vi "Parent Main Operation.vi"(8 "error in (no error)":errorcluster, 11 "Node Actor in":refnum<class "Node Actor.lvclass">) -> (0 "error out":errorcluster, 3 "Node Actor out":refnum<class "Node Actor.lvclass">)   [LabVIEW 2024, in "Node Actor.lvclass"]
uses:
  Node Actor.lvclass
  Message/Message.lvclass/Message.ctl
  Message/Public Data/Read CMD Type.vi
  Message/Message.lvclass
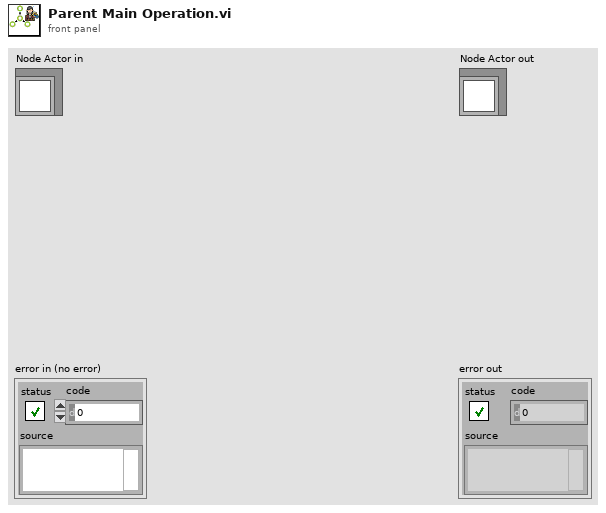
[diagram p1: front panel]
types:
  T1 = typedef "CMD Type.ctl" = enum16{"None", "General CMD", "1st CMD", "2nd CMD", "3rd CMD", "4th CMD", "5th CMD", "6th CMD", "7th CMD"}
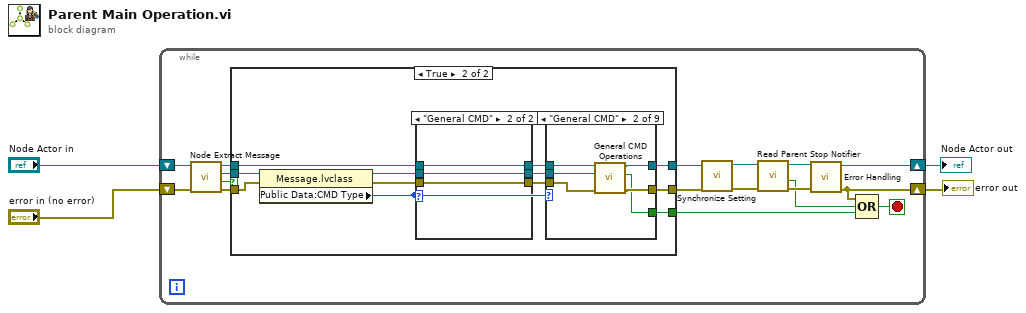
[diagram p0: block diagram]
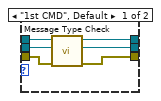
[diagram p3: hidden frame]
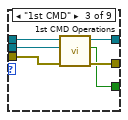
[diagram p5: hidden frame]
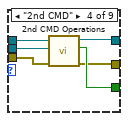
[diagram p6: hidden frame]
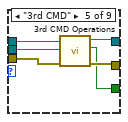
[diagram p7: hidden frame]
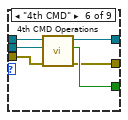
[diagram p8: hidden frame]
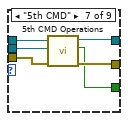
[diagram p9: hidden frame]
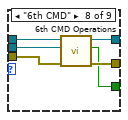
[diagram p10: hidden frame]
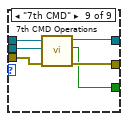
[diagram p11: hidden frame]
diagram:
  n1 = while {
    shift-right: [w13] -> w2
    shift-left: "Node Actor in" -> [w20]
    shift-right: [w6] -> w1
    shift-left: "error in (no error)" -> [w19]
    stop <- w21 stop-if-true
    n2 = call-dynamic "Node Extract Message.vi"("error in (no error)"=w19, "Node Actor in"=w20) -> ("error out"=w16:errorcluster, "Valid"=w14:bool, "Message Out"=w17:refnum<class "Message.lvclass">, "Node Actor out"=w18:refnum<class "Node Actor.lvclass">)  [unwired: 6 in]
    n3 = case shown="True" w14 {
      tunnel: [w22 w35] -> w11
      tunnel: w18 -> [w23 w27]
      tunnel: w17 -> [_ w32]
      tunnel: w16 -> [w22 w31]
      tunnel: [w23 w34] -> w12
      tunnel: [_ w33] -> w15
      frame False {
      }
      frame True {
        n4 = property class="Message.lvclass"(reference=w32, error in=w31) -> (reference out=w29:refnum<class "Message.lvclass">, error out=w28:errorcluster, "Public Data:CMD Type"=w30:T1)
        n5 = case shown="\"General CMD\"" w30 {
          tunnel: w29 -> [w40 w43]
          tunnel: w28 -> [w39 w42]
          tunnel: w27 -> [w41 w44]
          tunnel: [w36 w44] -> w26
          tunnel: [w37 w43] -> w25
          tunnel: [w38 w42] -> w24
          frame "1st CMD", Default {
            n6 = call-dynamic "Message Type Check.vi"("error in (no error)"=w39, "Message In"=w40, "System Actor in"=w41) -> ("error out"=w38:errorcluster, "Message Out"=w37:refnum<class "Message.lvclass">, "System Actor out"=w36:refnum<class "Node Actor.lvclass">)  [unwired: 6 in]
          }
          frame "General CMD" {
          }
        }
        n7 = case shown="\"General CMD\"" w30 {
          tunnel: w25 -> [_ w51 w57 w60 w69 w75 w81 w87 w93]
          tunnel: w26 -> [w46 w52 w58 w64 w70 w76 w82 w88 w94]
          tunnel: [w46 w48 w54 w63 w66 w73 w78 w85 w90] -> w34
          tunnel: w24 -> [w45 w50 w56 w59 w68 w74 w80 w86 w92]
          tunnel: [w45 w49 w55 w61 w67 w71 w79 w84 w91] -> w35
          tunnel: [_ w47 w53 w62 w65 w72 w77 w83 w89] -> w33
          frame "None", Default {
          }
          frame "General CMD" {
            n8 = call-dynamic "General CMD Operations.vi"("error in (no error)"=w50, "Message In"=w51, "System Actor in"=w52) -> ("error out"=w49:errorcluster, "Stop"=w47:bool, "System Actor out"=w48:refnum<class "Node Actor.lvclass">)  [unwired: 6 in]
          }
          frame "1st CMD" {
            n9 = call-dynamic "1st CMD Operations.vi"("error in (no error)"=w56, "Message In"=w57, "Node Actor in"=w58) -> ("error out"=w55:errorcluster, "Stop"=w53:bool, "Node Actor out"=w54:refnum<class "Node Actor.lvclass">)  [unwired: 6 in]
          }
          frame "2nd CMD" {
            n10 = call-dynamic "2nd CMD Operations.vi"("error in (no error)"=w59, "Message In"=w60, "System Actor in"=w64) -> ("error out"=w61:errorcluster, "Stop"=w62:bool, "System Actor out"=w63:refnum<class "Node Actor.lvclass">)  [unwired: 6 in]
          }
          frame "3rd CMD" {
            n11 = call-dynamic "3rd CMD Operations .vi"("error in (no error)"=w68, "Message In"=w69, "System Actor in"=w70) -> ("error out"=w67:errorcluster, "Stop"=w65:bool, "System Actor out"=w66:refnum<class "Node Actor.lvclass">)  [unwired: 6 in]
          }
          frame "4th CMD" {
            n12 = call-dynamic "4th CMD Operations.vi"("error in (no error)"=w74, "Message In"=w75, "System Actor in"=w76) -> ("error out"=w71:errorcluster, "Stop"=w72:bool, "System Actor out"=w73:refnum<class "Node Actor.lvclass">)  [unwired: 6 in]
          }
          frame "5th CMD" {
            n13 = call-dynamic "5th CMD Operations.vi"("error in (no error)"=w80, "Message In"=w81, "System Actor in"=w82) -> ("error out"=w79:errorcluster, "Stop"=w77:bool, "System Actor out"=w78:refnum<class "Node Actor.lvclass">)  [unwired: 6 in]
          }
          frame "6th CMD" {
            n14 = call-dynamic "6th CMD Operations .vi"("error in (no error)"=w86, "Message In"=w87, "System Actor in"=w88) -> ("error out"=w84:errorcluster, "Stop"=w83:bool, "System Actor out"=w85:refnum<class "Node Actor.lvclass">)  [unwired: 6 in]
          }
          frame "7th CMD" {
            n15 = call-dynamic "7th CMD Operations.vi"("error in (no error)"=w92, "Message In"=w93, "System Actor in"=w94) -> ("error out"=w91:errorcluster, "Stop"=w89:bool, "System Actor out"=w90:refnum<class "Node Actor.lvclass">)  [unwired: 6 in]
          }
        }
      }
    }
    n16 = call-dynamic "Synchronize Setting.vi"("error in (no error)"=w11, "Node Actor in"=w12) -> ("error out"=w8:errorcluster, "Node Actor out"=w10:refnum<class "Node Actor.lvclass">)  [unwired: 8 in]
    n17 = call-dynamic "Read Parent Stop Notifier.vi"("error in (no error)"=w8, "Node Actor in"=w10) -> ("error out"=w7:errorcluster, "Stop"=w5:bool, "Node Actor out"=w9:refnum<class "Node Actor.lvclass">)  [unwired: 7 in]
    n18 = call-dynamic "Error Handling.vi"("error in (no error)"=w7, "System Actor in"=w9) -> ("error out"=w6:errorcluster, "System Actor out"=w13:refnum<class "Node Actor.lvclass">)  [unwired: 8 in]
    n19 = Compound Arithmetic op=OR(w6, w5, w15) -> (w21:bool)
  }
  "error out" <- w1
  "Node Actor out" <- w2
